vi "WFGConfigureTriggerSingleCh.vi"(0 "object in":refnum<class "AD2_WFG_SDK.lvclass">, 2 "Ch":T1={"idxChannel"=0, "Settings out of range"=FALSE, "Carrier"={"Frequency (Hz)"=1000.0, "Amplitude (V)"=1.0, "Offset(V)"=0.0, "Symmetry(%) "=50.0, "Phase(Deg)"=0.0, "Function"=1, "Enable"=FALSE}, "Trigger"={"secRun(0=Cont)"=0.0, "secWait"=0.0, "cRepeat(0=inf)"=0, "Repeat Trigger"=FALSE, "TrigrSrc"=enum."trigrsrcNone"}, "FM Mod"={"Frequency (Hz)"=1000.0, "Amplitude (%)"=1.0, "Offset(V)"=0.0, "Symmetry(%) "=50.0, "Phase(Deg)"=0.0, "Function 2"=1, "Enable"=FALSE}} {"FM Mod"."Function 2" items=["DC"=0, "Sine"=1, "Square"=2, "Triangle"=3, "RampUp"=4, "RampDown"=5, "Noise"=6, "Pulse"=7, "Custom"=30]; "Carrier"."Function" items=["DC"=0, "Sine"=1, "Square"=2, "Triangle"=3, "RampUp"=4, "RampDown"=5, "Noise"=6, "Pulse"=7, "Custom"=30]}, 5 "error in (no error)":errorcluster) -> (14 "object out":refnum<class "AD2_WFG_SDK.lvclass">, 19 "error out":errorcluster)   [LabVIEW 2021, in "AD2_WFG_SDK.lvclass"]
uses:
  AD2_WFG_SDK.lvclass
  WFGCh.ctl
  AD2TriggerSources.ctl
  AD2_WFG_SDK.lvclass/AD2_WFG_SDK.ctl
  Olasdwf/Olasdwf.lvlib
  AD2_SDK_class/AD2_SDK.lvclass
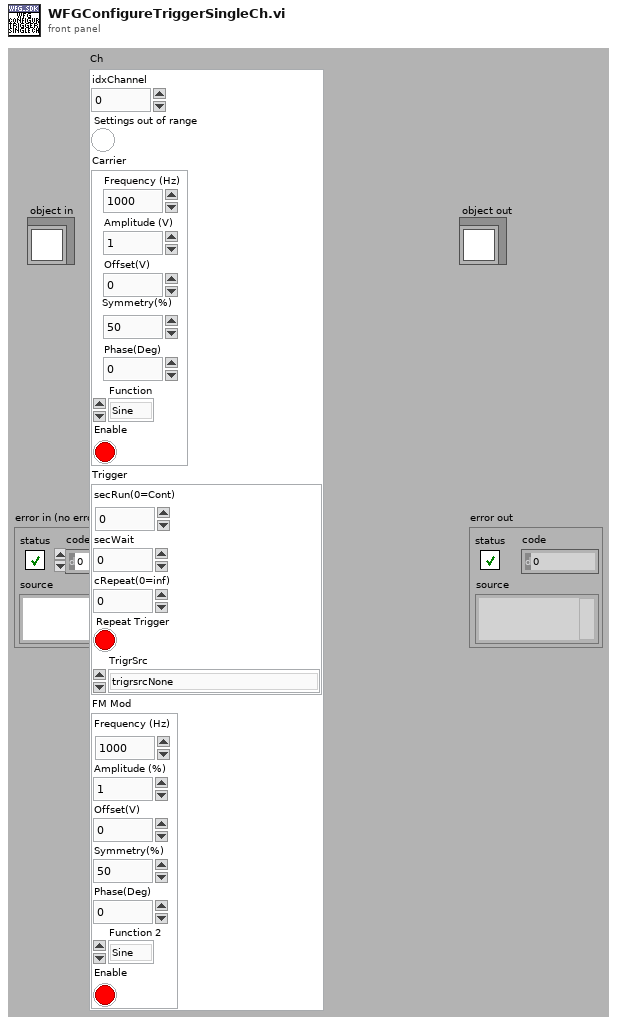
[diagram p1: front panel]
types:
  T1 = typedef "AD2_WFG_SDK.lvclass/WFGCh.ctl" = cluster{"idxChannel":i32, "Settings out of range":bool, "Carrier":cluster{"Frequency (Hz)":dbl, "Amplitude (V)":dbl, "Offset(V)":dbl, "Symmetry(%) ":dbl, "Phase(Deg)":dbl, "Function":u16, "Enable":bool}, "Trigger":cluster{"secRun(0=Cont)":dbl, "secWait":dbl, "cRepeat(0=inf)":i32, "Repeat Trigger":bool, "TrigrSrc":T2}, "FM Mod":cluster{"Frequency (Hz)":dbl, "Amplitude (%)":dbl, "Offset(V)":dbl, "Symmetry(%) ":dbl, "Phase(Deg)":dbl, "Function 2":u16, "Enable":bool}}
  T2 = typedef "AD2_SDK.lvclass/AD2TriggerSources.ctl" = enum8{"trigrsrcNone", "trigsrcPC", "trigsrcDetectorAnalogIn", "trigsrcDetectorDigitalIn", "trigsrcAnalogIn", "trigsrcDigitalIn", "trigsrcDigitalOut", "trigsrcAnalogOut1", "trigsrcAnalogOut2", "trigsrcAnalogOut3", "trigsrcAnalogOut4", "trigsrcExternal1", "trigsrcExternal2", "trigsrcExternal3", "trigsrcExternal4", ""}
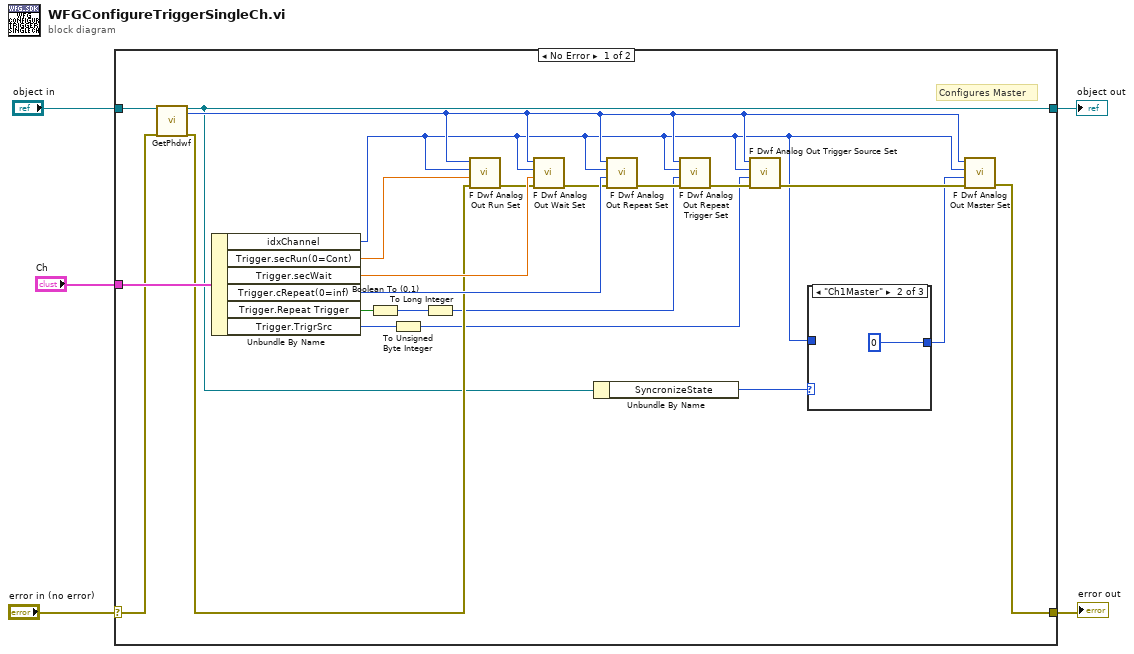
[diagram p0: block diagram]
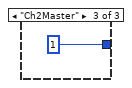
[diagram p3: hidden frame]
diagram:
  n1 = case shown="No Error" "error in (no error)" {
    selector: "error in (no error)" -> [w26 w33]
    tunnel: [w11 w33] -> w4
    tunnel: [w9 w32] -> w2
    tunnel: "object in" -> [w25 w32]
    tunnel: "Ch" -> [w28 _]
    frame No Error {
      # "Configures Master"
      n2 = call-dynamic "GetPhdwf.vi"("object in"=w25, "error in (no error)"=w26) -> ("object out"=w9:refnum<class "AD2_WFG_SDK.lvclass">, "phdwf"=w10:i32, "error out"=w19:errorcluster)  [unwired: 15 in]
      n3 = Unbundle By Name(w28) -> ("idxChannel"=w7:i32, "Trigger.secRun(0=Cont)"=w27:dbl, "Trigger.secWait"=w24:dbl, "Trigger.cRepeat(0=inf)"=w23:i32, "Trigger.Repeat Trigger"=w18:bool, "Trigger.TrigrSrc"=w14:T2)
      n4 = Boolean To (0,1)(Boolean=w18) -> (0, 1=w17:i16)
      n5 = To Unsigned Byte Integer(number=w14) -> (unsigned 8bit integer=w13:u8)
      n6 = To Long Integer(number=w17) -> (32bit integer=w16:i32)
      n7 = call "F Dwf Analog Out Run Set.vi"("error in (no error)"=w19, "secRun"=w27, "idxChannel"=w7, "hdwf"=w10) -> ("error out"=w22:errorcluster)  [unwired: 6 in, 1 out]
      n8 = call "F Dwf Analog Out Wait Set.vi"("error in (no error)"=w22, "secWait"=w24, "idxChannel"=w7, "hdwf"=w10) -> ("error out"=w21:errorcluster)  [unwired: 6 in, 1 out]
      n9 = Unbundle By Name(w9) -> ("SyncronizeState"=w8:enum16{"Independent", "Ch1Master", "Ch2Master"})
      n10 = call "F Dwf Analog Out Repeat Set.vi"("error in (no error)"=w21, "cRepeat"=w23, "idxChannel"=w7, "hdwf"=w10) -> ("error out"=w20:errorcluster)  [unwired: 6 in, 1 out]
      n11 = call "F Dwf Analog Out Repeat Trigger Set.vi"("error in (no error)"=w20, "fRepeatTrigger"=w16, "idxChannel"=w7, "hdwf"=w10) -> ("error out"=w15:errorcluster)  [unwired: 6 in, 1 out]
      n12 = call "F Dwf Analog Out Trigger Source Set.vi"("error in (no error)"=w15, "trigsrc"=w13, "idxChannel"=w7, "hdwf"=w10) -> ("error out"=w12:errorcluster)  [unwired: 6 in, 1 out]
      n13 = case shown="\"Ch1Master\"" w8 {
        tunnel: w7 -> [w29 _ _]
        tunnel: [w29 0 ("idxChannel") 1 ("idxChannel")] -> w6
        frame "Independent", Default {
        }
        frame "Ch1Master" {
        }
        frame "Ch2Master" {
        }
      }
      n14 = call "F Dwf Analog Out Master Set.vi"("error in (no error)"=w12, "idxMaster"=w6, "idxChannel"=w7, "hdwf"=w10) -> ("error out"=w11:errorcluster)  [unwired: 6 in, 1 out]
    }
    frame Error {
    }
  }
  "error out" <- w4
  "object out" <- w2
